vi "printHtmlWithIE.vi"(8 "error in (no error)":errorcluster, 11 "path to HTML":string) -> (0 "error out":errorcluster)   [LabVIEW 2017, in "LabVIEW NPOI.lvlib" / "MS-Excel.lvclass"]
uses:
  MS-Excel.lvclass
panel:
  in  "Automation Refnum in":refnum<k7>(container)
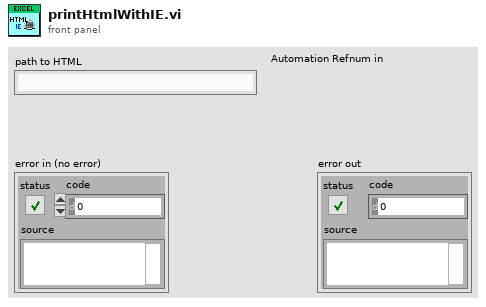
[diagram p1: front panel]
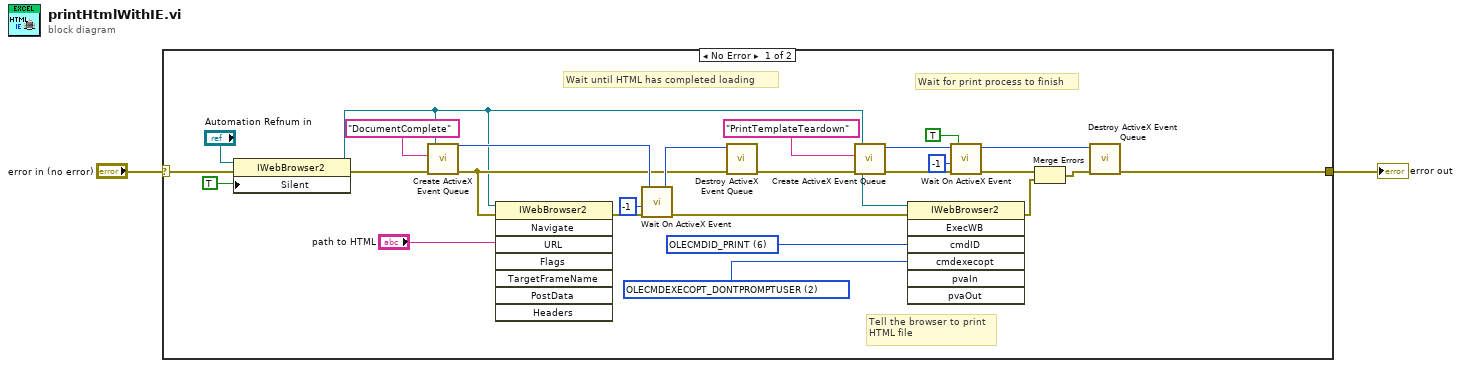
[diagram p0: block diagram]
diagram:
  n1 = case shown="No Error" "error in (no error)" {
    selector: "error in (no error)" -> [w16 w29]
    tunnel: [w7 w29] -> w2
    frame No Error {
      w26 = 2 items=["OLECMDEXECOPT_DODEFAULT", "OLECMDEXECOPT_PROMPTUSER", "OLECMDEXECOPT_DONTPROMPTUSER", "OLECMDEXECOPT_SHOWHELP"] ("cmdexecopt")
      w27 = 6 items=["OLECMDID_OPEN"=1, "OLECMDID_NEW"=2, "OLECMDID_SAVE"=3, "OLECMDID_SAVEAS"=4, "OLECMDID_SAVECOPYAS"=5, "OLECMDID_PRINT"=6, "OLECMDID_PRINTPREVIEW"=7, "OLECMDID_PAGESETUP"=8, "OLECMDID_SPELL"=9, "OLECMDID_PROPERTIES"=10, "OLECMDID_CUT"=11, "OLECMDID_COPY"=12, "OLECMDID_PASTE"=13, "OLECMDID_PASTESPECIAL"=14, "OLECMDID_UNDO"=15, "OLECMDID_REDO"=16, "OLECMDID_SELECTALL"=17, "OLECMDID_CLEARSELECTION"=18, "OLECMDID_ZOOM"=19, "OLECMDID_GETZOOMRANGE"=20, "OLECMDID_UPDATECOMMANDS"=21, "OLECMDID_REFRESH"=22, "OLECMDID_STOP"=23, "OLECMDID_HIDETOOLBARS"=24, "OLECMDID_SETPROGRESSMAX"=25, "OLECMDID_SETPROGRESSPOS"=26, "OLECMDID_SETPROGRESSTEXT"=27, "OLECMDID_SETTITLE"=28, "OLECMDID_SETDOWNLOADSTATE"=29, "OLECMDID_STOPDOWNLOAD"=30, "OLECMDID_ONTOOLBARACTIVATED"=31, "OLECMDID_FIND"=32, "OLECMDID_DELETE"=33, "OLECMDID_HTTPEQUIV"=34, "OLECMDID_HTTPEQUIV_DONE"=35, "OLECMDID_ENABLE_INTERACTION"=36, "OLECMDID_ONUNLOAD"=37, "OLECMDID_PROPERTYBAG2"=38, "OLECMDID_PREREFRESH"=39, "OLECMDID_SHOWSCRIPTERROR"=40, "OLECMDID_SHOWMESSAGE"=41, "OLECMDID_SHOWFIND"=42, "OLECMDID_SHOWPAGESETUP"=43, "OLECMDID_SHOWPRINT"=44, "OLECMDID_CLOSE"=45, "OLECMDID_ALLOWUILESSSAVEAS"=46, "OLECMDID_DONTDOWNLOADCSS"=47] ("cmdID")
      # "Wait for print process to finish"
      # "Tell the browser to print\nHTML file"
      # "Wait until HTML has completed loading"
      n2 = property class="IWebBrowser2"(reference="Automation Refnum in", error in=w16, "Silent"=TRUE) -> (reference out=w14:refnum<k7>, error out=w28:errorcluster)
      n3 = call <vilib>:"Create ActiveX Event Queue.vi"("error in (no error)"=w28, "Event Name"="DocumentComplete", "Automation Refnum"=w14) -> ("error out"=w19:errorcluster, "Event Queue"=w24:i32)  [unwired: 1 in, 2 out]
      n4 = invoke class="IWebBrowser2" method="Navigate"(reference=w14, error in=w19, "URL"="path to HTML") -> (error out=w20:errorcluster)  [unwired: 5 in, 7 out]
      n5 = call <vilib>:"Wait On ActiveX Event.vi"("error in (no error)"=w20, "ms Timeout (-1)"=-1 ("ms timeout (-1)"), "Event Queue"=w24) -> ("error out"=w18:errorcluster, "Event Queue Out"=w23:i32)  [unwired: 1 in, 2 out]
      n6 = call <vilib>:"Destroy ActiveX Event Queue.vi"("error in (no error)"=w19, "Event Queue"=w23) -> ("error out"=w12:errorcluster)  [unwired: 5 out]
      n7 = call <vilib>:"Create ActiveX Event Queue.vi"("error in (no error)"=w12, "Event Name"="PrintTemplateTeardown", "Automation Refnum"=w14) -> ("error out"=w5:errorcluster, "Event Queue"=w10:i32)  [unwired: 1 in, 2 out]
      n8 = invoke class="IWebBrowser2" method="ExecWB"(reference=w14, error in=w18, "cmdID"=w27, "cmdexecopt"=w26) -> (error out=w3:errorcluster)  [unwired: 3 in, 6 out]
      n9 = call <vilib>:"Wait On ActiveX Event.vi"("error in (no error)"=w5, "ms Timeout (-1)"=-1 ("ms timeout (-1)"), "Ignore Previous(T)"=TRUE, "Event Queue"=w10) -> ("error out"=w8:errorcluster, "Event Queue Out"=w9:i32)  [unwired: 2 out]
      n10 = Merge Errors(w8, w3) -> (w4:errorcluster)
      n11 = call <vilib>:"Destroy ActiveX Event Queue.vi"("error in (no error)"=w4, "Event Queue"=w9) -> ("error out"=w7:errorcluster)  [unwired: 5 out]
    }
    frame Error {
    }
  }
  "error out" <- w2
